vi "Change Snake Color Status.vi"(8 "error in (no error)":errorcluster, 11 "Snake in":refnum<class "Snake.lvclass">) -> (0 "error out":errorcluster, 3 "Snake out":refnum<class "Snake.lvclass">)   [LabVIEW 2021, in "Snake.lvclass"]
uses:
  Snake.lvclass
  C:/Users/poche/Programs/LabVIEW/Imposible_Snake/GameEl_class/GameEl.lvclass
  Snake.lvclass/Snake.ctl
  GameEl_class/GameEl.lvclass/GameEl.ctl
  GameEl_class/GameEl.lvclass
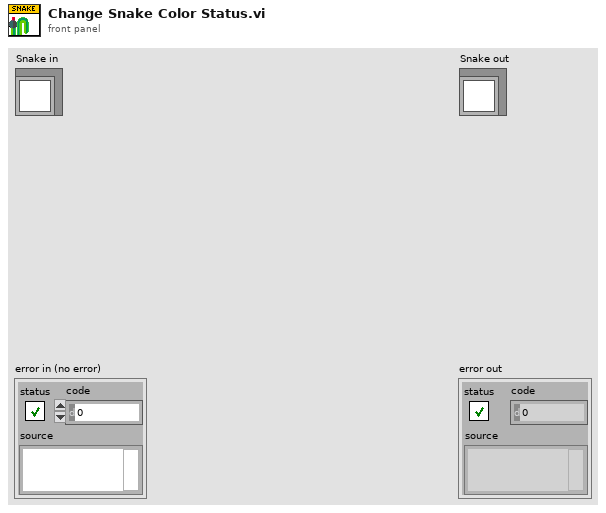
[diagram p1: front panel]
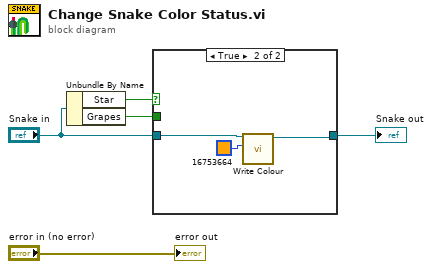
[diagram p0: block diagram]
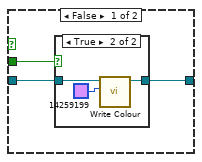
[diagram p2: hidden frame]
diagram:
  n1 = Unbundle By Name("Snake in") -> ("Star"=w1:bool, "Grapes"=w2:bool)
  n2 = case shown="True" w1 {
    tunnel: "Snake in" -> [w8 w14]
    tunnel: [w7 w13] -> w3
    tunnel: w2 -> [w6 _]
    frame False {
      n3 = case shown="True" w6 {
        tunnel: w8 -> [w9 w12]
        tunnel: [w9 w11] -> w7
        frame False {
        }
        frame True {
          n4 = call "Write Colour.vi"("Colour"=u32 14259199, "GameEl in"=w12) -> ("GameEl out"=w11:refnum<class "Snake.lvclass">)  [unwired: 8 in, 1 out]
        }
      }
    }
    frame True {
      n5 = call "Write Colour.vi"("Colour"=u32 16753664, "GameEl in"=w14) -> ("GameEl out"=w13:refnum<class "Snake.lvclass">)  [unwired: 8 in, 1 out]
    }
  }
  "Snake out" <- w3
  "error out" <- "error in (no error)"
